vi "DelFromXYGraphCurves.vi"(8 "error in (no error)":errorcluster caption="entrée d'erreur (pas d'erreur)", 9 "CurvIndex":i32, 10 "GraphIndex":i32, 11 "Interface en entrée":refnum<class "Interface.lvclass"> caption="DNL_LabVIEW Object in") -> (0 "error out":errorcluster caption="sortie d'erreur", 3 "Interface en sortie":refnum<class "Interface.lvclass"> caption="DNL_LabVIEW Object out")   [LabVIEW 2019, in "Interface.lvclass"]
uses:
  Interface.lvclass
  Interface.lvclass/Interface.ctl
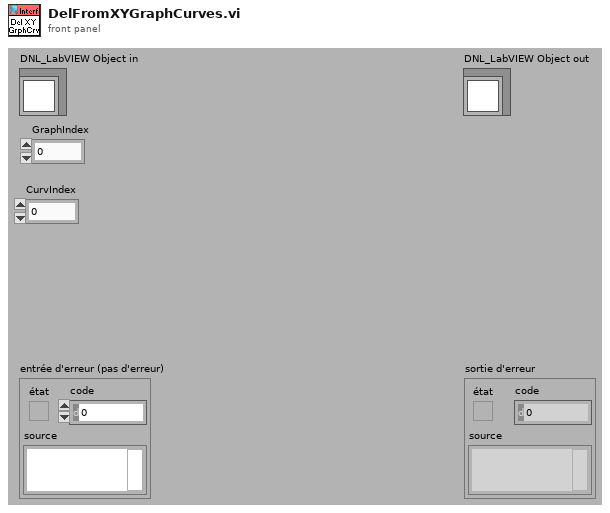
[diagram p1: front panel]
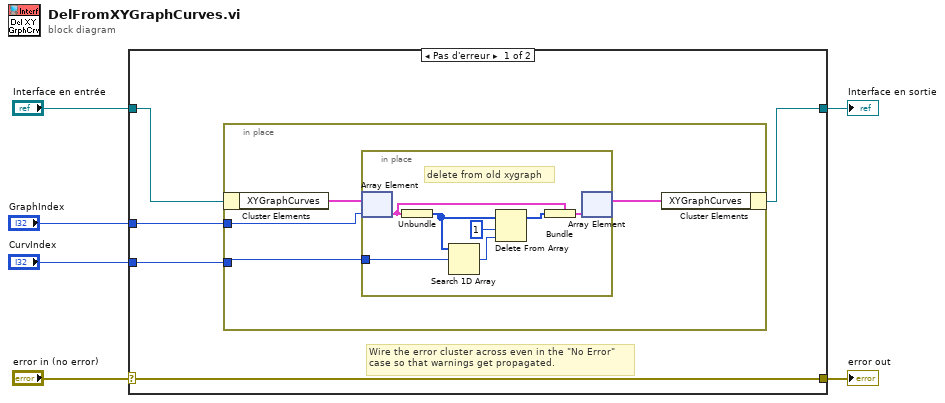
[diagram p0: block diagram]
diagram:
  n1 = case shown="Pas d'erreur" "error in (no error)" {
    selector: "error in (no error)" -> [w11 w24]
    tunnel: [w11 w24] -> w5
    tunnel: [w7 w23] -> w3
    tunnel: "Interface en entrée" -> [w10 w23]
    tunnel: "CurvIndex" -> [w9 _]
    tunnel: "GraphIndex" -> [w8 _]
    frame No Error {
      # "Wire the error cluster across even in the \"No Error\"\ncase so that warnings get propagated."
      n2 = in-place {
        in-place-border: w9 -> [w13]
        in-place-border: w8 -> [w14]
        n3 = in-place-cluster #1(w10) -> ("XYGraphCurves"=w15:cluster{"Tableau":i32[]}[])
        n4 = in-place {
          in-place-border: w13 -> [w16]
          # "delete from old xygraph"
          n5 = in-place-array #2(w15, w14) -> (w19:cluster{"Tableau":i32[]})
          n6 = Unbundle(w19) -> ("Tableau"=w20:i32[])
          n7 = Search 1D Array(1D array=w20, element=w16) -> (index of element=w21:i32)  [unwired: 1 in]
          n8 = Delete From Array(array=w20, length=1 ("longueur"), index=w21) -> (array with subset deleted=w17:i32[])  [unwired: 1 out]
          n9 = Bundle(cluster=w19, "Tableau"=w17) -> (w18:cluster{"Tableau":i32[]})
          n10 = in-place-array #2(w18) -> (w12:cluster{"Tableau":i32[]}[])  [unwired: 1 out]
        }
        n11 = in-place-cluster #1("XYGraphCurves"=w12) -> (w7:refnum<class "Interface.lvclass">)
      }
    }
    frame Error {
    }
  }
  "error out" <- w5
  "Interface en sortie" <- w3
